vi "BigIntIsSame.vi"(1 "b":cluster{"Boolean":bool, "Array":u64[]}, 2 "a":cluster{"Boolean":bool, "Array":u64[]}) -> (0 "a = b":bool)   [LabVIEW 2023]
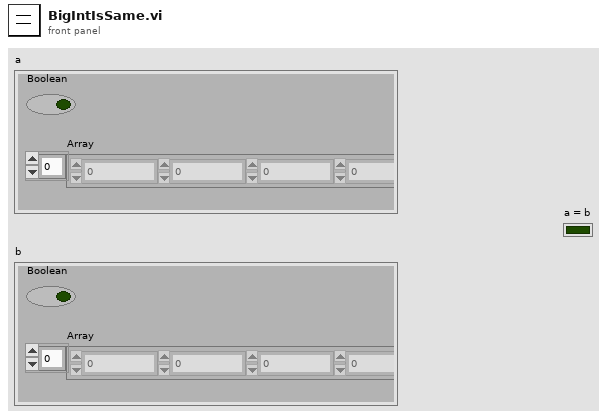
[diagram p1: front panel]
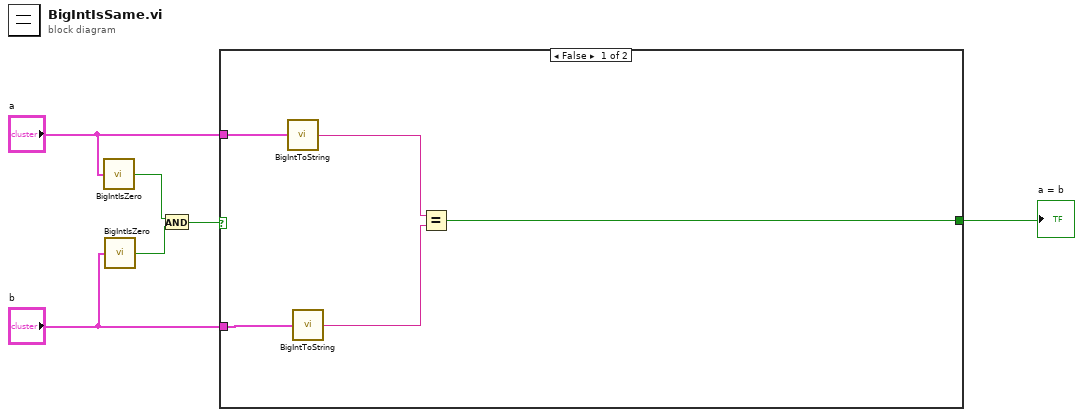
[diagram p0: block diagram]
diagram:
  n1 = call "BigIntIsZero.vi"("a"="a") -> ("a = 0"=w6:bool)
  n2 = call "BigIntIsZero.vi"("a"="b") -> ("a = 0"=w5:bool)
  n3 = And(x=w6, y=w5) -> (x .and. y?=w4:bool)
  n4 = case shown="False" w4 {
    selector: w4 -> [_ w12]
    tunnel: [w7 w12] -> w1
    tunnel: "a" -> [w11 _]
    tunnel: "b" -> [w10 _]
    frame False {
      n5 = call "BigIntToString.vi"("a"=w11) -> ("String"=w9:string)
      n6 = call "BigIntToString.vi"("a"=w10) -> ("String"=w8:string)
      n7 = Equal?(x=w9, y=w8) -> (x = y?=w7:bool)
    }
    frame True {
    }
  }
  "a = b" <- w1
